vi "Move to IR 2.vi"(0 "SS Index (3)":i32=3, 4 "Timeout (ms)":u32=3000, 5 "Drive 2":cluster{T1, T1}, 6 "Signal Strength":u8=115, 7 "Drive 1":cluster{T1, T1}, 8 "Direction":i16=7, 9 "Power/Speed 2":i8, 10 "Power/Speed 1":i8, 11 "NXT In":T2) -> (1 "Data Logging":cluster{i32, i32, "32bit integer":i32}[](array[cluster]), 3 "NXT Out":T2)   [LabVIEW 2012]
uses:
  <vilib>/NXT/Subs/LVHSConnector.ctl
  <vilib>/NXT/NXTIO Xnodes/NXTIOXNode/NXTIO.xnode
  <vilib>/NXT/Block Support/NXT_InputPort.ctl
  <vilib>/NXT/HiTechnic/HiTechnic Controls/HiTechnic Port.ctl
  <vilib>/NXT/LegoClasses/BrickReference/BrickReference.lvclass
  <vilib>/NXT/Hardware/Plugins/Open Port/OpenPortAddress.ctl
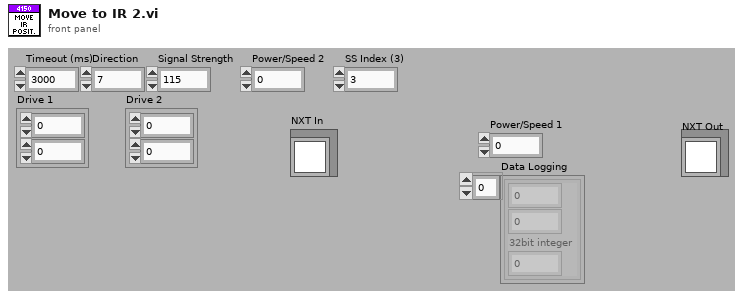
[diagram p1: front panel]
types:
  T1 = typedef "OpenPortAddress.ctl" = i32
  T2 = typedef "LVHSConnector.ctl" = refnum<class "BrickReference.lvclass">
  T3 = typedef "HiTechnic Port.ctl" = cluster{"Port":T4, "MUX Port":u8}
  T4 = typedef "NXT_InputPort.ctl" = u8
  T5 = cluster{"Direction (0-9)":i16, "Signal Strength (Array)":u8[]}
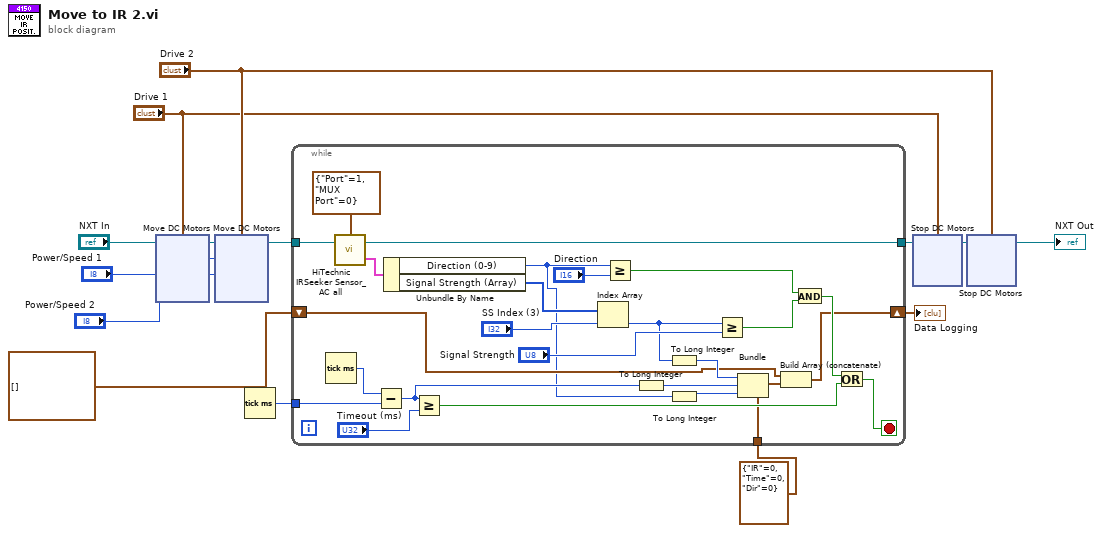
[diagram p0: block diagram]
diagram:
  n1 = xnode "Move DC Motors"("Power/Speed 2"="Power/Speed 2", "Power/Speed 1"="Power/Speed 1", "Motors"="Drive 1", "NXT"="NXT In") -> ("NXT"=w9:T2)
  n2 = xnode "Move DC Motors"("Power/Speed 2"="Power/Speed 2", "Power/Speed 1"="Power/Speed 1", "Motors"="Drive 2", "NXT"=w9) -> ("NXT"=w11:T2)
  n3 = Tick Count (ms)() -> (millisecond timer value=w12:u32)
  n4 = while {
    tunnel: w11 -> [w40]
    tunnel: w12 -> [w31]
    tunnel: [w27] -> w13
    shift-right: [w24] -> w4
    shift-left: cluster{"IR":i32, "Time":i32, "Dir":i32}[] [] -> [w18]
    tunnel: cluster{"IR":i32, "Time":i32, "Dir":i32} {"IR"=0, "Time"=0, "Dir"=0} -> [w15]
    stop <- w26 stop-if-true
    n5 = Tick Count (ms)() -> (millisecond timer value=w32:u32)
    n6 = call <vilib>:"HiTechnic IRSeeker Sensor_AC all.vi"("NXT"=w40, "Port/MUX"=T3 {"Port"=1, "MUX Port"=0}) -> ("All Info"=w39:T5, "NXT"=w27:T2)  [unwired: 1 in]
    n7 = Subtract(x=w32, y=w31) -> (x-y=w22:u32)
    n8 = Unbundle By Name(w39) -> ("Direction (0-9)"=w16:i16, "Signal Strength (Array)"=w37:u8[])
    n9 = Greater Or Equal?(x=w22, y="Timeout (ms)") -> (x >= y?=w28:bool)
    n10 = Index Array(array=w37, index="SS Index (3)") -> (element=w23:u8)
    n11 = Greater Or Equal?(x=w16, y="Direction") -> (x >= y?=w34:bool)
    n12 = To Long Integer(number=w22) -> (32bit integer=w21:i32)
    n13 = To Long Integer(number=w23) -> (32bit integer=w20:i32)
    n14 = To Long Integer(number=w16) -> (32bit integer=w17:i32)
    n15 = Greater Or Equal?(x=w23, y="Signal Strength") -> (x >= y?=w33:bool)
    n16 = Bundle(cluster=w15, "IR"=w20, "Time"=w21, "Dir"=w17) -> (w19:cluster{"IR":i32, "Time":i32, "Dir":i32})
    n17 = Build Array (concatenate)(w18, w19) -> (w24:cluster{"IR":i32, "Time":i32, "Dir":i32}[])
    n18 = And(x=w34, y=w33) -> (x .and. y?=w29:bool)
    n19 = Or(x=w29, y=w28) -> (x .or. y?=w26:bool)
  }
  "Data Logging" <- w4
  n20 = xnode "Stop DC Motors"("Motors"="Drive 1", "NXT"=w13) -> ("NXT"=w14:T2)
  n21 = xnode "Stop DC Motors"("Motors"="Drive 2", "NXT"=w14) -> ("NXT"=→"NXT Out":T2)
